vi "HFRR ADV v05 new software.vi"() -> ()   [LabVIEW 2025] (continued)
              }
              frame True {
                w1615 = FALSE ("FRICVALZ")
                n1291 = local write "FRICVALZ 3"(w1615) -> ()
                n1292 = local write "FRICVALZ 2"(w1615) -> ()
                n1293 = local write "FRICVALZ 4"(w1615) -> ()
                "FRICVALZ" <- w1616
              }
            }
            n1294 = Not A Number/Path/Refnum?(number/path/refnum=w1609) -> (NaN/Path/Refnum?=w1608:bool)
            n1295 = Not A Number/Path/Refnum?(number/path/refnum=w1605) -> (NaN/Path/Refnum?=w1607:bool)
            n1296 = Divide(x=w1605, y=1.96) -> (x/y=w1602:dbl)
            n1297 = Compound Arithmetic op=OR(w1608, w1607) -> (w1606:bool)
            n1298 = Not A Number/Path/Refnum?(number/path/refnum=w1602) -> (NaN/Path/Refnum?=w1603:bool)
            n1299 = case shown="True" w1606 {
              frame False {
              }
              frame True {
                n1300 = local write "TEMP"(0.0 ("TEMP")) -> ()
                n1301 = local write "FF 2"(0.0 ("FF 2")) -> ()
                n1302 = local write "reinit"(TRUE ("reinit")) -> ()
              }
            }
            n1303 = Select(t=0.0, s=w1603, f=w1602) -> (s? t:f=w1593:dbl)
            "COF 2" <- w1593
            n1304 = local write "COF 3"(w1593) -> ()
          }
        }
      }
    }
    n1305 = Wait (ms)(milliseconds to wait=u32 50) -> ()  [unwired: 1 out]
    n1306 = local read "Quit"() -> (w1531:bool)
    "Rate" <- 2500.0 ("No of Samples")
  }
  n1307 = while {
    tunnel: w57 -> [_]
    tunnel: [w1643] -> _
    tunnel: [w1619] -> w56
    i -> [w1643]
    stop <- w1619 stop-if-true
    # "C:\\LAB-IQ-NXT\\Scar View.exe"
    n1308 = local read "OK Button 16"() -> (w1632:bool)
    n1309 = local read "Main Tab"() -> (w1625:T2)
    n1310 = local read "service 3"() -> (w1626:bool)
    n1311 = local read "OPEN 6"() -> (w1628:bool)
    n1312 = local read "EDIT 2"() -> (w1630:bool)
    n1313 = flat-sequence {
      frame #0 {
        n1314 = local read "SAVE 2"() -> (w2245:bool)
        n1315 = stacked-sequence {
          frame #0 {
            n1316 = local read "EDIT"() -> (w2299:bool)
            n1317 = case shown="True" w2299 {
              tunnel: [u8 2 ("Disabled") u8 0 ("Disabled")] -> _
              frame False {
                w2301 = FALSE
                n1318 = local write "Password"("") -> ()
                n1319 = property on="SrvM CP" class="Bool (strict)"("Visible"=w2301) -> ()  [unwired: 2 in, 2 out]
                n1320 = property on="message" class="Str"("Visible"=w2301) -> ()  [unwired: 2 in, 2 out]
                n1321 = local write "x = y?"(w2301) -> ()
                n1322 = property on="Password" class="Str"("Visible"=w2301) -> ()  [unwired: 2 in, 2 out]
                n1323 = property on="ENTER THE NEW PASSWORD" class="Str"("Visible"=w2301) -> ()  [unwired: 2 in, 2 out]
                n1324 = property on="ENTER CURRENT PASSWORD" class="Str"("Visible"=w2301) -> ()  [unwired: 2 in, 2 out]
                n1325 = local write "SrvM CP"(w2301) -> ()
              }
              frame True {
                w2304 = TRUE
                n1326 = property on="SrvM CP" class="Bool (strict)"("Visible"=w2304) -> ()  [unwired: 2 in, 2 out]
                n1327 = property on="Password" class="Str"("Visible"=w2304) -> ()  [unwired: 2 in, 2 out]
              }
            }
            "dipl pwd" <- "@143$\n" ("dipl pwd")
          }
          frame #1 {
            # "Gain password"
            n1328 = String To Byte Array(string="ENTER CURRENT PASSWORD") -> (unsigned byte array=w2309:u8[])
            n1329 = Search 1D Array(1D array=w2309, element=u8 10) -> (index of element=w2312:i32)  [unwired: 1 in]
            n1330 = Index Array(array=w2309, index=w2312) -> (element=w2308:u8)
            n1331 = Equal?(x=w2308, y=10) -> (x = y?=w2306:bool)
            n1332 = case shown="True" w2306 {
              frame False {
                n1333 = property on="ENTER THE NEW PASSWORD" class="Str"("Visible"=FALSE) -> ()  [unwired: 2 in, 2 out]
              }
              frame True {
                # "password"
                # "change password logic"
                n1334 = local read "ENTER CURRENT PASSWORD"() -> (w2325:string)
                n1335 = local read "dipl pwd"() -> (w2319:string)
                n1336 = String To Byte Array(string=w2325) -> (unsigned byte array=w2327:u8[])
                n1337 = String To Byte Array(string=w2319) -> (unsigned byte array=w2320:u8[])
                n1338 = Array Size(array=w2327) -> (size(s)=w2324:i32)
                n1339 = Array Size(array=w2320) -> (size(s)=w2322:i32)
                n1340 = for {
                  N: w2324 -> [_]
                  tunnel: w2327 -> [w2351]
                  tunnel: [w2349] -> w2328 mode=indexing
                  tunnel: w2324 -> [w2343]
                  i -> [w2344]
                  n1341 = Decrement(x=w2343) -> (x-1=w2341:i32)
                  n1342 = Equal?(x=w2344, y=w2341) -> (x = y?=w2342:bool)
                  n1343 = Index Array(array=w2351, index=w2344) -> (element=w2345:u8)
                  n1344 = Number To Decimal String(number=w2345) -> (decimal integer string=w2350:string)  [unwired: 1 in]
                  n1345 = Select(t="", s=w2342, f="\r") -> (s? t:f=w2347:string)
                  n1346 = Concatenate Strings(w2350, w2347) -> (w2349:string)
                }
                n1347 = for {
                  N: w2322 -> [_]
                  tunnel: w2320 -> [w2339]
                  tunnel: [w2337] -> w2321 mode=indexing
                  tunnel: w2322 -> [w2334]
                  i -> [w2335]
                  n1348 = Decrement(x=w2334) -> (x-1=w2333:i32)
                  n1349 = Equal?(x=w2335, y=w2333) -> (x = y?=w2332:bool)
                  n1350 = Index Array(array=w2339, index=w2335) -> (element=w2338:u8)
                  n1351 = Number To Decimal String(number=w2338) -> (decimal integer string=w2336:string)  [unwired: 1 in]
                  n1352 = Select(t="", s=w2332, f="\r") -> (s? t:f=w2329:string)
                  n1353 = Concatenate Strings(w2336, w2329) -> (w2337:string)
                }
                n1354 = local read "string"() -> (w2326:string)
                n1355 = Concatenate Strings(w2321) -> (w2315:string)
                n1356 = Concatenate Strings(w2326) -> (w2323:string)
                n1357 = Concatenate Strings(w2328) -> (w2316:string)
                n1358 = Equal?(x=w2316, y=w2323) -> (x = y?=w2318:bool)
                n1359 = Equal?(x=w2316, y=w2315) -> (x = y?=w2314:bool)
                n1360 = Or(x=w2318, y=w2314) -> (x .or. y?=w2317:bool)
                n1361 = case shown="True" w2317 {
                  frame False {
                  }
                  frame True {
                    n1362 = property on="ENTER THE NEW PASSWORD" class="Str"("Visible"=TRUE) -> ()  [unwired: 2 in, 2 out]
                  }
                }
              }
            }
          }
          frame #2 {
            n1363 = String To Byte Array(string="ENTER THE NEW PASSWORD") -> (unsigned byte array=w2354:u8[])
            n1364 = Search 1D Array(1D array=w2354, element=u8 10) -> (index of element=w2358:i32)  [unwired: 1 in]
            n1365 = Index Array(array=w2354, index=w2358) -> (element=w2356:u8)
            n1366 = Equal?(x=w2356, y=10) -> (x = y?=w2353:bool)
            n1367 = case shown="False" w2353 {
              frame False {
              }
              frame True {
                n1368 = local write "EDIT"(FALSE) -> ()
                n1369 = local write "SrvM CP"(FALSE) -> ()
                n1370 = local read "ENTER THE NEW PASSWORD"() -> (w2361:string)
                n1371 = String To Byte Array(string=w2361) -> (unsigned byte array=w2366:u8[])
                n1372 = Array Size(array=w2366) -> (size(s)=w2363:i32)
                n1373 = for {
                  N: w2363 -> [_]
                  tunnel: w2366 -> [w2379]
                  tunnel: [w2376] -> w2368 mode=indexing
                  tunnel: w2363 -> [w2371]
                  i -> [w2369]
                  n1374 = Decrement(x=w2371) -> (x-1=w2372:i32)
                  n1375 = Equal?(x=w2369, y=w2372) -> (x = y?=w2373:bool)
                  n1376 = Index Array(array=w2379, index=w2369) -> (element=w2378:u8)
                  n1377 = Number To Decimal String(number=w2378) -> (decimal integer string=w2377:string)  [unwired: 1 in]
                  n1378 = Select(t="", s=w2373, f="\r") -> (s? t:f=w2370:string)
                  n1379 = Concatenate Strings(w2377, w2370) -> (w2376:string)
                }
                n1380 = local read "file path"() -> (w2360:path)
                n1381 = Concatenate Strings(w2368) -> (w2362:string)
                n1382 = Delete(path (use dialog)=w2360) -> (deleted path=w2364:path)  [unwired: 4 in, 2 out]
                n1383 = call <vilib>:"Write Characters To File.vi"("append to file? (new file:F)"=FALSE, "character string"=w2362, "file path (dialog if empty)"=w2364) -> ()  [unwired: 2 in, 1 out]
              }
            }
          }
          frame #3 {
            n1384 = case shown="True" "SrvM CP" {
              frame False {
                w2382 = ""
                n1385 = local write "ENTER CURRENT PASSWORD"(w2382) -> ()
                n1386 = local write "ENTER THE NEW PASSWORD"(w2382) -> ()
                n1387 = property on="ENTER CURRENT PASSWORD" class="Str"("Visible"=FALSE) -> ()  [unwired: 2 in, 2 out]
              }
              frame True {
                n1388 = property on="ENTER THE NEW PASSWORD" class="Str"() -> ("Visible"=w2383:bool)  [unwired: 2 in, 2 out]
                n1389 = Not(x=w2383) -> (.not. x?=w2384:bool)
                n1390 = property on="ENTER CURRENT PASSWORD" class="Str"("Visible"=w2384) -> ()  [unwired: 2 in, 2 out]
              }
            }
          }
          frame #4 {
            n1391 = String To Byte Array(string="Password") -> (unsigned byte array=w2391:u8[])
            n1392 = Search 1D Array(1D array=w2391, element=u8 10) -> (index of element=w2389:i32)  [unwired: 1 in]
            n1393 = Index Array(array=w2391, index=w2389) -> (element=w2390:u8)
            n1394 = Equal?(x=w2390, y=10) -> (x = y?=w2386:bool)
            n1395 = case shown="True" w2386 {
              frame False {
              }
              frame True {
                # "password"
                # "password"
                n1396 = local read "Password"() -> (w2404:string)
                n1397 = String To Byte Array(string=w2404) -> (unsigned byte array=w2407:u8[])
                n1398 = String To Byte Array(string="@143$\n") -> (unsigned byte array=w2393:u8[])
                n1399 = Array Size(array=w2407) -> (size(s)=w2402:i32)
                n1400 = Array Size(array=w2393) -> (size(s)=w2398:i32)
                n1401 = for {
                  N: w2402 -> [_]
                  tunnel: w2407 -> [w2441]
                  tunnel: [w2439] -> w2408 mode=indexing
                  tunnel: w2402 -> [w2436]
                  i -> [w2437]
                  n1402 = Decrement(x=w2436) -> (x-1=w2435:i32)
                  n1403 = Index Array(array=w2441, index=w2437) -> (element=w2440:u8)
                  n1404 = Equal?(x=w2437, y=w2435) -> (x = y?=w2434:bool)
                  n1405 = Number To Decimal String(number=w2440) -> (decimal integer string=w2438:string)  [unwired: 1 in]
                  n1406 = Select(t="", s=w2434, f="\r") -> (s? t:f=w2431:string)
                  n1407 = Concatenate Strings(w2438, w2431) -> (w2439:string)
                }
                n1408 = for {
                  N: w2398 -> [_]
                  tunnel: w2393 -> [w2452]
                  tunnel: [w2450] -> w2396 mode=indexing
                  tunnel: w2398 -> [w2447]
                  i -> [w2448]
                  n1409 = Decrement(x=w2447) -> (x-1=w2446:i32)
                  n1410 = Index Array(array=w2452, index=w2448) -> (element=w2451:u8)
                  n1411 = Equal?(x=w2448, y=w2446) -> (x = y?=w2445:bool)
                  n1412 = Number To Decimal String(number=w2451) -> (decimal integer string=w2449:string)  [unwired: 1 in]
                  n1413 = Select(t="", s=w2445, f="\r") -> (s? t:f=w2442:string)
                  n1414 = Concatenate Strings(w2449, w2442) -> (w2450:string)
                }
                n1415 = local read "file path"() -> (w2392:path)
                n1416 = call <vilib>:"Read Characters From File.vi"("file path (dialog if empty)"=w2392) -> ("character string"=w2406:string)  [unwired: 5 in, 3 out]
                "string" <- w2406
                n1417 = flat-sequence {
                  tunnel: [w2409] -> w2403
                  frame #0 {
                    w2409 = ""
                    n1418 = local write "Password"(w2409) -> ()
                  }
                }
                n1419 = Concatenate Strings(w2396) -> (w2397:string)
                n1420 = Concatenate Strings(w2406) -> (w2405:string)
                n1421 = Concatenate Strings(w2408) -> (w2400:string)
                n1422 = Equal?(x=w2400, y=w2405) -> (x = y?=w2395:bool)
                n1423 = Equal?(x=w2400, y=w2397) -> (x = y?=w2401:bool)
                n1424 = Or(x=w2395, y=w2401) -> (x .or. y?=w2394:bool)
                "x = y?" <- w2394
                n1425 = case shown="True" w2394 {
                  selector: w2394 -> [w2411 _]
                  tunnel: w2403 -> [_ _]
                  frame False {
                    n1426 = And(x=w2411, y=TRUE ("Visible")) -> (x .and. y?=w2412:bool)
                    n1427 = property on="message" class="Str"("Visible"=w2412) -> ()  [unwired: 2 in, 2 out]
                  }
                  frame True {
                    n1428 = control-ref of="This VI"() -> (w2423:refnum<vi>)
                    n1429 = property class="VI"(reference=w2423) -> (reference out=w2414:refnum<vi>, error out=w2418:errorcluster, "Panel"=w2422:refnum<vi>)  [unwired: 1 in]
                    n1430 = property on="message" class="Str"("Visible"=FALSE) -> ()  [unwired: 2 in, 2 out]
                    n1431 = property class="Pnl"(reference=w2422, error in=w2418) -> (reference out=w2416:refnum<vi>, error out=w2419:errorcluster, "Panes[]"=w2421:refnum<vi>[])
                    n1432 = for {
                      tunnel: w2421 -> [w2430] mode=indexing
                      tunnel: T15."Always On" ("Horizontal Scrollbar Visibility") -> [w2429]
                      tunnel: w2419 -> [w2426]
                      tunnel: [w2425] -> w2417
                      n1433 = property class="Pane"(reference=w2430, error in=w2426, "HorizScrollbarVisibility"=w2429) -> (reference out=w2427:refnum<vi>, error out=w2428:errorcluster)
                      n1434 = Close Reference(reference=w2427, error in (no error)=w2428) -> (error out=w2425:errorcluster)
                    }
                    n1435 = Close Reference(reference=w2416, error in (no error)=w2417) -> (error out=w2415:errorcluster)
                    n1436 = Close Reference(reference=w2414, error in (no error)=w2415) -> (error out=→"error out 6":errorcluster)
                  }
                }
              }
            }
          }
        }
        n1437 = local read "x = y?"() -> (w2251:bool)
        n1438 = local read "HUMIDITY: 2"() -> (w2253:dbl)
        n1439 = local read "HUMIDITY:"() -> (w2252:dbl)
        n1440 = property on="Port 2 Error" class="Clust (strict)"("Visible"="EDIT") -> ()  [unwired: 2 in, 2 out]
        n1441 = property on="Port 1 Error" class="Clust (strict)"("Visible"="EDIT") -> ()  [unwired: 2 in, 2 out]
        n1442 = case shown="True" "SrvM CP 2" {
          frame False {
          }
          frame True {
            n1443 = local write "SrvM CP 2"(FALSE ("SrvM CP 2")) -> ()
            n1444 = local read "HUMIDITY: 2"() -> (w2292:dbl)
            n1445 = local read "TEMP INTERCEPT: 2"() -> (w2291:dbl)
            n1446 = local read "DISPLACEMENT : 4"() -> (w2295:dbl)
            n1447 = local read "TEMPERATURE : 2"() -> (w2294:dbl)
            n1448 = local read "STROKE GAIN : 2"() -> (w2296:dbl)
            n1449 = local read "FRIC. FORCE : 2"() -> (w2297:dbl)
            n1450 = local read "AIR TEMP INTERCEPT: 2"() -> (w2290:dbl)
            n1451 = local read "AIR TEMPERATURE : 2"() -> (w2293:dbl)
            n1452 = local write "HUMIDITY:"(w2292) -> ()
            n1453 = local write "AIR TEMP INTERCEPT:"(w2291) -> ()
            n1454 = local write "TEMPERATURE :"(w2294) -> ()
            n1455 = local write "FRIC. FORCE :"(w2297) -> ()
            n1456 = local write "STROKE GAIN :"(w2296) -> ()
            n1457 = local write "DISPLACEMENT :"(w2295) -> ()
            n1458 = local write "AIR TEMPERATURE :"(w2293) -> ()
            n1459 = local write "TEMP INTERCEPT:"(w2290) -> ()
          }
        }
        n1460 = Or(x="SAVE", y=w2245) -> (x .or. y?=w2246:bool)
        n1461 = And(x="EDIT", y=w2251) -> (x .and. y?=w2249:bool)
        n1462 = local read "DISPLACEMENT : 4"() -> (w2262:dbl)
        n1463 = local read "TEMPERATURE : 2"() -> (w2260:dbl)
        n1464 = local read "STROKE GAIN : 2"() -> (w2266:dbl)
        n1465 = local read "DISPLACEMENT :"() -> (w2261:dbl)
        n1466 = local read "FRIC. FORCE : 2"() -> (w2269:dbl)
        n1467 = local read "TEMPERATURE :"() -> (w2258:dbl)
        n1468 = local read "STROKE GAIN :"() -> (w2265:dbl)
        n1469 = local read "FRIC. FORCE :"() -> (w2268:dbl)
        n1470 = case shown="True" w2249 {
          tunnel: [u8 2 ("Disabled") u8 0 ("Disabled")] -> w2248
          tunnel: [w2613 TRUE ("Visible")] -> w2247
          frame False {
            w2613 = FALSE ("Visible")
            n1471 = local write "EDIT 2"(w2613) -> ()
          }
          frame True {
          }
        }
        n1472 = case shown="True" w2246 {
          frame False {
          }
          frame True {
            n1473 = stacked-sequence {
              seq-local: [w2461 _ _] -> [_ w2608 _]
              frame #0 {
                (unwired) i16 5 ("precision (6)")
                # "[CH1]    - FF\n[CH2]   - TEMPERATURE\n[CH3]    - Humidity\n[CH4]    - AIR TEMP\n[CH5]\\- Visa Uno\n[CH6] \\- Visa Due\n[CH7]  \\- file path\n[CH8]   - Displacement Gain\n[CHA]   - Stroke Gain\n[CHB]   - Stroke PID Gain\n[CHC]   -Language Selection\n[CHD]   -Power +\n[CHE]   -Power_\n[CHF]   -Heater\n[CHG]   -Humidity Wet\n[CHH]   -Humidity Dry\n[CHI]   -Integral Time"
                n1474 = local read "Language Selection"() -> (w2509:enum16{"English", "Russian"})
                n1475 = local read "CH-HUMIDITY WET"() -> (w2467:u16)
                n1476 = local read "CH-HUMIDITY DRY"() -> (w2464:u16)
                n1477 = local read "STROKE GAIN :"() -> (w2453:dbl)
                n1478 = local read "CH-POWER +"() -> (w2476:u16)
                n1479 = local read "CH-POWER -"() -> (w2473:u16)
                n1480 = local read "CH-HEATER"() -> (w2470:u16)
                n1481 = local read "AIR TEMPERATURE :"() -> (w2456:dbl)
                n1482 = local read "DISPLACEMENT :"() -> (w2454:dbl)
                n1483 = local read "TEMPERATURE :"() -> (w2457:dbl)
                n1484 = local read "FRIC. FORCE :"() -> (w2458:dbl)
                n1485 = local read "HUMIDITY:"() -> (w2455:dbl)
                n1486 = Path To String(path="File Path") -> (string=w2525:string)
                n1487 = Number To Fractional String(number=w2453, width (-)=i16 10 ("precision (6)"), precision (6)=i16 5) -> (F-format string=w2516:string)  [unwired: 1 in]
                n1488 = Number To Fractional String(number=w2509, width (-)=i16 10 ("precision (6)"), precision (6)=i16 5) -> (F-format string=w2505:string)  [unwired: 1 in]
                n1489 = Number To Fractional String(number=w2476, width (-)=i16 10 ("precision (6)"), precision (6)=i16 5) -> (F-format string=w2499:string)  [unwired: 1 in]
                n1490 = Number To Fractional String(number=w2473, width (-)=i16 10 ("precision (6)"), precision (6)=i16 5) -> (F-format string=w2496:string)  [unwired: 1 in]
                n1491 = Number To Fractional String(number=w2470, width (-)=i16 10 ("precision (6)"), precision (6)=i16 5) -> (F-format string=w2491:string)  [unwired: 1 in]
                n1492 = Number To Fractional String(number=w2467, width (-)=i16 10 ("precision (6)"), precision (6)=i16 5) -> (F-format string=w2488:string)  [unwired: 1 in]
                n1493 = Number To Fractional String(number=w2464, width (-)=i16 10 ("precision (6)"), precision (6)=i16 5) -> (F-format string=w2483:string)  [unwired: 1 in]
                n1494 = local read "Com Port 1"() -> (w2460:refnum<visa-resource-name>)
                n1495 = local read "Com Port 2"() -> (w2459:refnum<visa-resource-name>)
                n1496 = Concatenate Strings(w2525, "\\" ("string")) -> (w2524:string)
                n1497 = Number To Fractional String(number=w2458, width (-)=i16 10 ("precision (6)"), precision (6)=i16 5) -> (F-format string=w2557:string)  [unwired: 1 in]
                n1498 = Number To Fractional String(number=w2457, width (-)=i16 10 ("precision (6)"), precision (6)=i16 5) -> (F-format string=w2556:string)  [unwired: 1 in]
                n1499 = Number To Fractional String(number=w2455, width (-)=i16 10 ("precision (6)"), precision (6)=i16 5) -> (F-format string=w2550:string)  [unwired: 1 in]
                n1500 = Number To Fractional String(number=w2456, width (-)=i16 10 ("precision (6)"), precision (6)=i16 5) -> (F-format string=w2544:string)  [unwired: 1 in]
                n1501 = Number To Fractional String(number=w2454, width (-)=i16 10 ("precision (6)"), precision (6)=i16 5) -> (F-format string=w2517:string)  [unwired: 1 in]
                n1502 = Concatenate Strings("[CHA]" ("string"), w2516, "- Stroke Gain" ("string"), "\r") -> (w2510:string)
                n1503 = Concatenate Strings("[CHC]" ("string"), w2505, "-Language Selection" ("string"), "\r") -> (w2502:string)
                n1504 = Concatenate Strings("[CHD]" ("string"), w2499, "-Power +" ("string"), "\r") -> (w2481:string)
                n1505 = Concatenate Strings("[CHG]" ("string"), w2488, "-Humidity Wet" ("string"), "\r") -> (w2478:string)
                n1506 = Concatenate Strings("[CHH]" ("string"), w2483, "-Humidity Dry" ("string"), "\r") -> (w2477:string)
                n1507 = Concatenate Strings("[CH1]" ("string"), w2557, " - FF" ("string"), "\r") -> (w2555:string)
                n1508 = Concatenate Strings("[CH2]" ("string"), w2556, " - TEMPERATURE" ("string"), "\r") -> (w2554:string)
                n1509 = Concatenate Strings("[CH3]" ("string"), w2550, " - Humidity" ("string"), "\r") -> (w2547:string)
                n1510 = Concatenate Strings("[CH4]" ("string"), w2544, " - AIR TEMP" ("string"), "\r") -> (w2540:string)
                n1511 = Concatenate Strings("[CH5]" ("string"), w2460, "- Visa Uno" ("string"), "\r") -> (w2533:string)
                n1512 = Concatenate Strings("[CH6]" ("string"), w2459, "- Visa Due" ("string"), "\r") -> (w2528:string)
                n1513 = Concatenate Strings("[CH7]" ("string"), w2524, "- file path" ("string"), "\r") -> (w2527:string)
                n1514 = Concatenate Strings("[CH8]" ("string"), w2517, "- Displacement Gain" ("string"), "\r") -> (w2520:string)
                n1515 = Concatenate Strings("[CHE]" ("string"), w2496, "-Power_" ("string"), "\r") -> (w2480:string)
                n1516 = Concatenate Strings("[CHF]" ("string"), w2491, "-Heater" ("string"), "\r") -> (w2479:string)
                n1517 = Concatenate Strings(w2555, w2554, w2547, w2540, w2533, w2528, w2527, w2520, w2510, w2502, w2481, w2480, w2479, w2478, w2477) -> (w2461:string)
                "gain" <- w2461
              }
              frame #1 {
                n1518 = local read "Camera Port :"() -> (w2569:string)
                n1519 = local read "C3 :"() -> (w2577:refnum<visa-resource-name>)
                n1520 = local read "TEMP INTERCEPT:"() -> (w2578:dbl)
                n1521 = local read "AIR TEMP INTERCEPT:"() -> (w2579:dbl)
                n1522 = Concatenate Strings("[CH8]" ("string"), w2569, "- Visa Camera" ("string"), "\r") -> (w2568:string)
                n1523 = Concatenate Strings("[CH7]" ("string"), w2577, "- Visa Humidity" ("string"), "\r") -> (w2573:string)
                n1524 = Number To Fractional String(number=w2578, width (-)=i16 10 ("precision (6)"), precision (6)=i16 5) -> (F-format string=w2596:string)  [unwired: 1 in]
                n1525 = local read "Com Port 3"() -> (w2580:refnum<visa-resource-name>)
                n1526 = Number To Fractional String(number=w2579, width (-)=i16 10 ("precision (6)"), precision (6)=i16 5) -> (F-format string=w2603:string)  [unwired: 1 in]
                n1527 = Concatenate Strings("[CHK]" ("string"), w2596, "-TEMP INTERCEPT" ("string"), "\r") -> (w2592:string)
                n1528 = Concatenate Strings("[SNO]" ("string"), "S.NO", "-" ("string"), "\r") -> (w2588:string)
                n1529 = Concatenate Strings("[CHJ]" ("string"), w2603, "-AIR TEMP INTERCEPT" ("string"), "\r") -> (w2593:string)
                n1530 = Concatenate Strings("[CHL]" ("string"), w2580, "- Visa humid" ("string"), "\r") -> (w2583:string)
                n1531 = String To Path(string="C:\\LAB-IQ\\calibrate WO 2465.dcf") -> (path=w2581:path)
                n1532 = Concatenate Strings(w2608, w2593, w2592, w2588, w2583, w2573, w2568) -> (w2607:string)
                n1533 = call <vilib>:"Write Characters To File.vi"("append to file? (new file:F)"=FALSE, "character string"=w2607, "file path (dialog if empty)"=w2581) -> ()  [unwired: 2 in, 1 out]
              }
              frame #2 {
                n1534 = local write "Lan flag"(0.0 ("Lan flag")) -> ()
                n1535 = local write "conststatus"(0.0 ("rpm value : 2")) -> ()
                n1536 = local write "SAVE"(FALSE ("OK Button 14")) -> ()
                n1537 = local write "SAVE 2"(FALSE ("SAVE 2")) -> ()
              }
            }
          }
        }
        n1538 = Subtract(x=w2253, y=w2252) -> (x-y=w2254:dbl)
        n1539 = local read "AIR TEMPERATURE : 2"() -> (w2257:dbl)
        n1540 = local read "AIR TEMPERATURE :"() -> (w2256:dbl)
        n1541 = Divide(x=w2254, y=w2252) -> (x/y=w2276:dbl)
        n1542 = Subtract(x=w2269, y=w2268) -> (x-y=w2267:dbl)
        n1543 = Subtract(x=w2260, y=w2258) -> (x-y=w2259:dbl)
        n1544 = Subtract(x=w2266, y=w2265) -> (x-y=w2264:dbl)
        n1545 = Subtract(x=w2262, y=w2261) -> (x-y=w2263:dbl)
        n1546 = Subtract(x=w2257, y=w2256) -> (x-y=w2255:dbl)
        n1547 = Divide(x=w2267, y=w2268) -> (x/y=w2287:dbl)
        n1548 = Divide(x=w2259, y=w2258) -> (x/y=w2280:dbl)
        n1549 = Divide(x=w2264, y=w2265) -> (x/y=w2284:dbl)
        n1550 = Divide(x=w2263, y=w2261) -> (x/y=w2283:dbl)
        n1551 = Multiply(x=w2276, y=100.0) -> (x*y=→"HUMIDITY  Calibration Error":dbl)
        n1552 = Divide(x=w2255, y=w2256) -> (x/y=w2279:dbl)
        n1553 = Multiply(x=w2287, y=100.0) -> (x*y=→"FRIC. FORCE Calibration Error":dbl)
        n1554 = Multiply(x=w2280, y=100.0) -> (x*y=→"TEMPERATURE  Calibration Error":dbl)
        n1555 = Multiply(x=w2284, y=100.0) -> (x*y=→"STROKE Calibration Error":dbl)
        n1556 = Multiply(x=w2283, y=100.0) -> (x*y=→"DISPLACEMENT  Calibration Error":dbl)
        n1557 = property on="EDIT 2" class="Bool (strict)"("Visible"=w2247) -> ()  [unwired: 2 in, 2 out]
        n1558 = property on="SAVE" class="Bool (strict)"("Visible"=w2247) -> ()  [unwired: 2 in, 2 out]
        n1559 = property on="SrvM CP" class="Bool (strict)"("Disabled"=w2248) -> ()  [unwired: 2 in, 2 out]
        n1560 = property on="visa due" class="CmbBox"("Disabled"=w2248) -> ()  [unwired: 2 in, 2 out]
        n1561 = property on="File Path" class="Path"("Disabled"=w2248) -> ()  [unwired: 2 in, 2 out]
        n1562 = Multiply(x=w2279, y=100.0) -> (x*y=→"AIR TEMPERATURE  Calibration Error":dbl)
        n1563 = property on="Language Selection" class="Enum (strict)"("Visible"=w2247) -> ()  [unwired: 2 in, 2 out]
        n1564 = property on="Tab Control 7" class="TabCtl (strict)"("Disabled"=w2248) -> ()  [unwired: 2 in, 2 out]
        n1565 = property on="AIR TEMP INTERCEPT:" class="DigNum (strict)"("Disabled"=w2248) -> ()  [unwired: 2 in, 2 out]
        n1566 = property on="CH-POWER -" class="DigNum (strict)"("Disabled"=w2248) -> ()  [unwired: 2 in, 2 out]
        n1567 = property on="CH-POWER +" class="DigNum (strict)"("Disabled"=w2248) -> ()  [unwired: 2 in, 2 out]
        n1568 = property on="AIR TEMPERATURE :" class="DigNum (strict)"("Disabled"=w2248) -> ()  [unwired: 2 in, 2 out]
        n1569 = property on="STROKE GAIN :" class="DigNum (strict)"("Disabled"=w2248) -> ()  [unwired: 2 in, 2 out]
        n1570 = property on="SPEED OUT:" class="DigNum (strict)"("Disabled"=w2248) -> ()  [unwired: 2 in, 2 out]
        n1571 = property on="CH-HUMIDITY DRY" class="DigNum (strict)"("Disabled"=w2248) -> ()  [unwired: 2 in, 2 out]
        n1572 = property on="HUMIDITY:" class="DigNum (strict)"("Disabled"=w2248) -> ()  [unwired: 2 in, 2 out]
        n1573 = property on="CH-HUMIDITY WET" class="DigNum (strict)"("Disabled"=w2248) -> ()  [unwired: 2 in, 2 out]
        n1574 = property on="TEMPERATURE :" class="DigNum (strict)"("Disabled"=w2248) -> ()  [unwired: 2 in, 2 out]
        n1575 = property on="DISPLACEMENT :" class="DigNum (strict)"("Disabled"=w2248) -> ()  [unwired: 2 in, 2 out]
        n1576 = property on="CH-HEATER" class="DigNum (strict)"("Disabled"=w2248) -> ()  [unwired: 2 in, 2 out]
        n1577 = property on="TEMP INTERCEPT:" class="DigNum (strict)"("Disabled"=w2248) -> ()  [unwired: 2 in, 2 out]
        n1578 = property on="FRIC. FORCE :" class="DigNum (strict)"("Disabled"=w2248) -> ()  [unwired: 2 in, 2 out]
      }
    }
    n1579 = local read "RUN"() -> (w1642:bool)
    n1580 = local read "RUN"() -> (w1640:bool)
    n1581 = disable-structure shown="Disabled" {
      disable-tunnel: [w1657 _] -> w1623
      disable-tunnel: [w1656 _] -> w1621
      frame Disabled {
        n1582 = local read "Temperature before test"() -> (w1650:dbl)
        n1583 = local read "Temperature after test"() -> (w1663:dbl)
        n1584 = case shown="True" "Save Results" {
          frame False {
          }
          frame True {
            w1679 = "\r"
            n1585 = local write "Save Results"(FALSE ("OK Button 5")) -> ()
            n1586 = local read "Temperature before test"() -> (w1717:dbl)
            n1587 = local read "Temperature after test"() -> (w1719:dbl)
            n1588 = local read "Humidity before test"() -> (w1716:dbl)
            n1589 = local read "Humidity after test"() -> (w1718:dbl)
            n1590 = local read "WS1.4"() -> (w1723:dbl)
            n1591 = local read "AVP"() -> (w1721:dbl)
            n1592 = Number To Fractional String(number=w1723, width (-)=i16 6, precision (6)=i16 1) -> (F-format string=w1683:string)  [unwired: 1 in]
            n1593 = local read "MWSD"() -> (w1720:dbl)
            n1594 = local read "String"() -> (w1712:string)
            n1595 = local read "FILE"() -> (w1715:string)
            n1596 = local read "HCF"() -> (w1722:dbl)
            n1597 = Number To Fractional String(number=w1716, width (-)=i16 6, precision (6)=i16 1) -> (F-format string=w1708:string)  [unwired: 1 in]
            n1598 = Number To Fractional String(number=w1717, width (-)=i16 6, precision (6)=i16 1) -> (F-format string=w1705:string)  [unwired: 1 in]
            n1599 = Number To Fractional String(number=w1718, width (-)=i16 6, precision (6)=i16 1) -> (F-format string=w1701:string)  [unwired: 1 in]
            n1600 = Number To Fractional String(number=w1719, width (-)=i16 6, precision (6)=i16 1) -> (F-format string=w1697:string)  [unwired: 1 in]
            n1601 = Number To Fractional String(number=w1721, width (-)=i16 6, precision (6)=i16 3) -> (F-format string=w1690:string)  [unwired: 1 in]
            n1602 = Concatenate Strings(w1712, w1715) -> (w1734:string)
            n1603 = Number To Fractional String(number=w1720, width (-)=i16 6, precision (6)=i16 1) -> (F-format string=w1694:string)  [unwired: 1 in]
            n1604 = Number To Fractional String(number=w1722, width (-)=i16 6, precision (6)=i16 2) -> (F-format string=w1688:string)  [unwired: 1 in]
            n1605 = Concatenate Strings("(" ("string"), w1683, ")Microns" ("string")) -> (w1682:string)
            n1606 = local read "REMARKS"() -> (w1714:string)
            "REMARKS 2" <- w1714
            n1607 = Concatenate Strings("(" ("string"), w1708, " ) % RH," ("string")) -> (w1709:string)
            n1608 = Concatenate Strings(w1688, ")" ("string")) -> (w1686:string)
            n1609 = Concatenate Strings("(" ("string"), w1705, ")  Deg C ," ("string")) -> (w1704:string)
            n1610 = Concatenate Strings("(" ("string"), w1701, " ) % RH," ("string")) -> (w1700:string)
            n1611 = Concatenate Strings("(" ("string"), w1697, ")  Deg C ," ("string")) -> (w1696:string)
            n1612 = Concatenate Strings("(" ("string"), w1694, ")  Microns," ("string")) -> (w1693:string)
            n1613 = Concatenate Strings("(" ("string"), w1690, ")  kPa," ("string")) -> (w1680:string)
            n1614 = Concatenate Strings(w1734, ".dwm" ("Substring")) -> (w1732:string)
            n1615 = String To Path(string=w1732) -> (path=w1731:path)
            n1616 = Concatenate Strings(w1714, w1679, " Humidity before test= " ("Substring"), w1709, w1679, " Temperature before test = " ("Substring"), w1704, w1679, " Humidity after test= " ("Substring"), w1700, w1679, "Temperature after test = " ("Substring"), w1696, w1679, "MSD = " ("Substring"), w1693, w1679, "  AVP = " ("Substring"), w1680, w1679, "  HCF                     =( " ("Substring"), w1686, w1679, " WS1.4                  = " ("Substring"), w1682, w1679) -> (w1678:string)
            "data" <- w1678
            n1617 = call <vilib>:"Write Characters To File.vi"("append to file? (new file:F)"=FALSE, "character string"=w1678, "file path (dialog if empty)"=w1731) -> ()  [unwired: 2 in, 1 out]
            n1618 = Match Pattern(string=w1678, regular expression="!") -> (after substring=→"export":string)  [unwired: 1 in, 3 out]
          }
        }
        n1619 = Add(x=231.864, y=w1650) -> (x+y=w1647:dbl)
        n1620 = Add(x=231.864, y=w1663) -> (x+y=w1660:dbl)
        n1621 = Divide(x=1705.984, y=w1647) -> (x/y=w1648:dbl)
        n1622 = Divide(x=1705.984, y=w1660) -> (x/y=w1661:dbl)
        n1623 = local read "Humidity before test"() -> (w1652:dbl)
        n1624 = local read "Humidity after test"() -> (w1665:dbl)
        n1625 = Subtract(x=8.017352 ("y"), y=w1648) -> (x-y=w1674:dbl)
        n1626 = Subtract(x=8.017352 ("y"), y=w1661) -> (x-y=w1668:dbl)
        n1627 = expression code="10**y"(w1674) -> (w1654:dbl)
        n1628 = expression code="10**y"(w1668) -> (w1667:dbl)
        n1629 = Multiply(x=w1652, y=w1654) -> (x*y=w1653:dbl)
        n1630 = Multiply(x=w1665, y=w1667) -> (x*y=w1666:dbl)
        n1631 = Divide(x=w1653, y=750.0) -> (x/y=w1669:dbl)
        n1632 = Divide(x=w1666, y=750.0) -> (x/y=w1670:dbl)
        n1633 = Add(x=w1669, y=w1670) -> (x+y=w1671:dbl)
        n1634 = Divide(x=w1671, y=2.0) -> (x/y=w1673:dbl)
        n1635 = local write "AVP"(w1673) -> ()
        n1636 = Subtract(x=1.4, y=w1673) -> (x-y=w1656:dbl)
        n1637 = local read "HCF"() -> (w1657:dbl)
      }
      frame Enabled {
      }
    }
    n1638 = case shown="True" "EDIT 3" {
      frame False {
      }
      frame True {
        n1639 = local write "EDIT 3"(FALSE ("EDIT 3")) -> ()
        n1640 = local write "Main Tab"(T2."About" ("Main Tab")) -> ()
      }
    }
    n1641 = case shown="False" w1642 {
      frame False {
        n1642 = local read "stopT"() -> (w2620:bool)
        n1643 = case shown="True" w2620 {
          frame False {
          }
          frame True {
            n1644 = local write "stopT"(FALSE) -> ()
          }
        }
      }
      frame True {
        "stopT" <- TRUE
      }
    }
    n1645 = case shown="False" w1640 {
      frame False {
      }
      frame True {
      }
    }
    n1646 = case shown="True" w1630 {
      frame False {
        n1647 = property on="Password 2" class="Str"("Visible"=FALSE) -> ()  [unwired: 2 in, 2 out]
        n1648 = local write "Password 2"("" ("Password")) -> ()
      }
      frame True {
        n1649 = property on="Password 2" class="Str"("Visible"=TRUE) -> ()  [unwired: 2 in, 2 out]
        n1650 = Equal?(x="Password 2", y="HFRR1234") -> (x = y?=w1762:bool)
        n1651 = case shown="True" w1762 {
          tunnel: "Password 2" -> [w1765 _]
          frame False {
            n1652 = String Length(string=w1765) -> (length=w1766:i32)
            n1653 = Greater Than 0?(x=w1766) -> (x > 0?=w1764:bool)
            n1654 = case shown="False" w1764 {
              frame False {
                n1655 = property on="Password 2" class="Str"("Caption.Text"="Password (Advance Setting)") -> ()  [unwired: 2 in, 2 out]
              }
              frame True {
                n1656 = property on="Password 2" class="Str"("Caption.Text"="Incorrect Password!") -> ()  [unwired: 2 in, 2 out]
              }
            }
          }
          frame True {
            n1657 = local write "EDIT 2"(FALSE ("EDIT 2")) -> ()
            n1658 = local write "Password 2"("" ("Password")) -> ()
            n1659 = local write "Main Tab"(T2."Advance" ("Main Tab")) -> ()
            n1660 = local write "Main Dashboard Buttons"(T1."Advance" ("Main Dashboard Buttons")) -> ()
          }
        }
      }
    }
    n1661 = case shown="True" "Prog Uno" {
      frame False {
      }
      frame True {
        n1662 = stacked-sequence {
          frame #0 {
            n1663 = Delete(path (use dialog)=path "C:/LAB-IQ-NXT/UNOCOMPILE.bat" ("working directory")) -> ()  [unwired: 4 in, 3 out]
          }
          frame #1 {
            n1664 = local read "Com Port 1"() -> (w2227:refnum<visa-resource-name>)
            n1665 = Concatenate Strings("cmd.exe /c \"mode " ("command line"), w2227, ":1200,n,8,1\"\n" ("command line")) -> (w2232:string)
            n1666 = Concatenate Strings(w2232, "CD\\\nCD WinDucom\navrdude -C avrdude.conf -v -patmega328p -carduino -P" ("command line"), w2227, " -b115200 -D -Uflash:w:UNO_V20.hex:i\n" ("command line"), "\r") -> (w2234:string)
            "STR" <- w2234
            n1667 = call <vilib>:"Write Characters To File.vi"("append to file? (new file:F)"=FALSE, "character string"=w2234, "file path (dialog if empty)"=path "C:/LAB-IQ/UNOCOMPILE.bat" ("working directory")) -> ()  [unwired: 2 in, 1 out]
          }
          frame #2 {
            n1668 = disable-structure shown="Disabled" {
              frame Disabled {
                w2238 = "cmd.exe  /c \"C:\\LAB-IQ-NXT\\UNOCOMPILE.bat\"" ("string")
                n1669 = local write "Prog Uno"(FALSE ("run minimized? (F)")) -> ()
                n1670 = call <vilib>:"System Exec.vi"("expected output size  (4096)"=u32 65535, "run minimized? (F)"=FALSE, "wait until completion? (T)"=TRUE ("run minimized? (F)"), "working directory"=path "C:/LAB-IQ-NXT", "standard input"=w2238, "command line"=w2238) -> ("error out"=w2237:errorcluster, "standard output"=→"String 42":string)  [unwired: 2 in, 2 out]
                "error out 3" <- w2237
                n1671 = flat-sequence {
                  tunnel: w2237 -> [_]
                  frame #0 {
                  }
                }
              }
              frame Enabled {
              }
            }
          }
        }
      }
    }
    n1672 = case shown="\"CEC F-096-A-06\"" "TEST STANDARD" {
      tunnel: [2.0 ("Set Temp") 0.0 ("Set Temp") 2.0 ("Set Temp") 0.0 ("Set Temp")] -> w1631
      frame "ASTM D6079", Default {
        w2184 = 50.0 ("Hz")
        w2185 = 53.0 ("Set Rh")
        w2187 = 1.0 ("Set Strk")
        w2186 = 60.0 ("Set Temp")
        # "astm hide"
        n1673 = local write "NORMAL LOAD"(200.0 ("NORMAL LOAD")) -> ()
        n1674 = local write "Set Strk"(w2187) -> ()
        n1675 = local write "Set Hz"(w2184) -> ()
        n1676 = local write "Set Temp"(w2186) -> ()
        n1677 = local write "Set Rh"(w2185) -> ()
        n1678 = local write "test time"(75.0 ("test time")) -> ()
        n1679 = local write "Set Stroke:"(w2187) -> ()
        n1680 = local write "Set Humidity:"(w2185) -> ()
        n1681 = local write "Set Frequency:"(w2184) -> ()
        n1682 = local write "Set Temperature:"(w2186) -> ()
        "Test Standard" <- "ASTM D6079" ("Test Standard 2")
      }
      frame "ISO 12156" {
        n1683 = local write "Set Strk"(1.0 ("Set Strk")) -> ()
        n1684 = local write "NORMAL LOAD"(200.0 ("NORMAL LOAD")) -> ()
        n1685 = local write "Set Temp"(60.0 ("Set Temp")) -> ()
        n1686 = local write "test time"(75.0 ("test time")) -> ()
        n1687 = local write "Set Hz"(50.0 ("Hz")) -> ()
        n1688 = local write "Set Rh"(53.0 ("Set Rh")) -> ()
      }
      frame "CEC F-096-A-06" {
        n1689 = local write "Set Strk"(1.0 ("Set Strk")) -> ()
        n1690 = local write "NORMAL LOAD"(200.0 ("NORMAL LOAD")) -> ()
        n1691 = local write "Set Temp"(60.0 ("Set Temp")) -> ()
        n1692 = local write "test time"(75.0 ("test time")) -> ()
        n1693 = local write "Set Hz"(50.0 ("Hz")) -> ()
        n1694 = local write "Set Rh"(53.0 ("Set Rh")) -> ()
      }
      frame "Custom" {
      }
    }
    n1695 = case shown="True" "Prog Due" {
      frame False {
      }
      frame True {
        n1696 = stacked-sequence {
          frame #0 {
            n1697 = Delete(path (use dialog)=path "C:/LAB-IQ/DUECOMPILE.bat" ("working directory")) -> ()  [unwired: 4 in, 3 out]
          }
          frame #1 {
            n1698 = disable-structure shown="Disabled" {
              frame Disabled {
                n1699 = local read "visa due"() -> (w2209:string)
                n1700 = Concatenate Strings("cmd.exe /c \"mode " ("command line"), w2209, ":1200,n,8,1\"\n" ("command line")) -> (w2214:string)
                n1701 = Concatenate Strings(w2214, "CD\\\nCD WinDucom\nTIMEOUT 1\n bossac.exe -i -d --port=" ("command line"), w2209, " -U false -e -w -v -b DUE.bin -R\n" ("command line"), "\r") -> (w2216:string)
                "concatenated string 2" <- w2216
                n1702 = call <vilib>:"Write Characters To File.vi"("append to file? (new file:F)"=FALSE, "character string"=w2216, "file path (dialog if empty)"=path "C:/LAB-IQ-NXT/DUECOMPILE.bat" ("working directory")) -> ()  [unwired: 2 in, 1 out]
              }
              frame Enabled {
              }
            }
          }
          frame #2 {
            # "C:\\LAB-IQ-NXT\\DUECOMPILE.bat"
            n1703 = disable-structure shown="Disabled" {
              frame Disabled {
                w2221 = "cmd.exe  /c \"C:\\LAB-IQ-NXT\\DUECOMPILE.bat\"" ("string")
                n1704 = call <vilib>:"System Exec.vi"("expected output size  (4096)"=u32 65535, "run minimized? (F)"=FALSE, "wait until completion? (T)"=TRUE ("run minimized? (F)"), "working directory"=path "C:/LAB-IQ-NXT", "standard input"=w2221, "command line"=w2221) -> ("error out"=w2220:errorcluster, "standard output"=→"String 44":string)  [unwired: 2 in, 2 out]
                "error out 4" <- w2220
                n1705 = flat-sequence {
                  tunnel: w2220 -> [_]
                  frame #0 {
                  }
                }
              }
              frame Enabled {
              }
            }
            n1706 = local write "Prog Due"(FALSE ("Prog Due")) -> ()
          }
        }
      }
    }
    n1707 = Or(x=w1628, y=w1626) -> (x .or. y?=w1627:bool)
    n1708 = case shown="\"About\"" w1625 {
      tunnel: [T20."Acquire" ("Main Tab") T20."Compare Files" ("Main Tab") T20."About" ("Main Tab")] -> w1638
      frame "Acquire", Default {
      }
      frame "Compare Files" {
      }
      frame "About" {
      }
    }
    n1709 = Or(x=w1632, y="OPEN") -> (x .or. y?=w1633:bool)
    n1710 = case shown="True" w1633 {
      tunnel: w1632 -> [_ w1773]
      frame False {
      }
      frame True {
        n1711 = stacked-sequence {
          tunnel: w1773 -> [_ w1840 _ _]
          frame #0 {
            w1789 = "  " ("String 6")
            n1712 = local write "OPEN"(FALSE ("open")) -> ()
            n1713 = local read "string1 2"() -> (w1777:string)
            n1714 = local read "string1 3"() -> (w1776:string)
            n1715 = local read "string1 4"() -> (w1775:string)
            n1716 = property on="OPEN" class="Bool (strict)"("Visible"=FALSE) -> ()  [unwired: 2 in, 2 out]
            n1717 = local write "String 6"(w1789) -> ()
            n1718 = local write "String 7"(w1789) -> ()
            n1719 = local write "String 8"(w1789) -> ()
            n1720 = local write "String 12"(w1789) -> ()
            n1721 = local read "OK Button 16"() -> (w1774:bool)
            n1722 = String To Path(string=w1777) -> (path=w1785:path)
            n1723 = String To Path(string=w1776) -> (path=w1784:path)
            n1724 = String To Path(string=w1775) -> (path=w1783:path)
            n1725 = case shown="True" w1774 {
              tunnel: [w1790 w1791] -> w1778
              frame False {
                n1726 = local read "string1"() -> (w1790:string)
              }
              frame True {
                n1727 = local read "String Indicator 4"() -> (w1791:string)
              }
            }
            n1728 = Open/Create/Replace File "Open File"(file path (use dialog)=w1785) -> (refnum out=w1781:refnum<file>)  [unwired: 5 in, 2 out]
            n1729 = Open/Create/Replace File "Open File"(file path (use dialog)=w1784) -> (refnum out=w1780:refnum<file>)  [unwired: 5 in, 2 out]
            n1730 = Open/Create/Replace File "Open File"(file path (use dialog)=w1783) -> (refnum out=w1779:refnum<file>)  [unwired: 5 in, 2 out]
            n1731 = while {
              tunnel: w1781 -> [w1803]
              i -> [w1799]
              stop <- w1798 continue-if-true
              (unwired) TRUE ("line mode (F)")
              n1732 = Read from Text File "Read File"(file (use dialog)=w1803) -> (text=w1800:string)  [unwired: 3 in, 3 out]
              n1733 = local write "Numeric 11"(w1799) -> ()
              n1734 = String Length(string=w1800) -> (length=w1802:i32)
              n1735 = Greater?(x=w1802, y=1) -> (0:w1798:bool)
            }
            n1736 = while {
              tunnel: w1780 -> [w1809]
              i -> [w1805]
              stop <- w1804 continue-if-true
              (unwired) TRUE ("line mode (F)")
              n1737 = Read from Text File "Read File"(file (use dialog)=w1809) -> (text=w1806:string)  [unwired: 3 in, 3 out]
              n1738 = local write "Numeric 12"(w1805) -> ()
              n1739 = String Length(string=w1806) -> (length=w1808:i32)
              n1740 = Greater?(x=w1808, y=1) -> (0:w1804:bool)
            }
            n1741 = while {
              tunnel: w1779 -> [w1815]
              i -> [w1811]
              stop <- w1810 continue-if-true
              (unwired) TRUE ("line mode (F)")
              n1742 = Read from Text File "Read File"(file (use dialog)=w1815) -> (text=w1812:string)  [unwired: 3 in, 3 out]
              n1743 = local write "Numeric 13"(w1811) -> ()
              n1744 = String Length(string=w1812) -> (length=w1814:i32)
              n1745 = Greater?(x=w1814, y=1) -> (0:w1810:bool)
            }
            n1746 = String To Path(string=w1778) -> (path=w1786:path)
            n1747 = Open/Create/Replace File "Open File"(file path (use dialog)=w1786) -> (refnum out=w1782:refnum<file>)  [unwired: 5 in, 2 out]
            n1748 = while {
              tunnel: w1782 -> [w1797]
              i -> [w1793]
              stop <- w1792 continue-if-true
              (unwired) TRUE ("line mode (F)")
              n1749 = Read from Text File "Read File"(file (use dialog)=w1797) -> (text=w1794:string)  [unwired: 3 in, 3 out]
              n1750 = local write "Numeric 8"(w1793) -> ()
              n1751 = String Length(string=w1794) -> (length=w1796:i32)
              n1752 = Greater?(x=w1796, y=1) -> (0:w1792:bool)
            }
          }
          frame #1 {
            w1967 = FALSE ("ACTUAL   MERGE")
            # "Sample Temp"
            # "ECR"
            # "COF"
            # "Time\nCOF\nFF\nTemp"
            n1753 = case shown="True" w1840 {
              tunnel: [w1987 w1988] -> w1841
              frame False {
                n1754 = local read "string1"() -> (w1987:string)
              }
              frame True {
                n1755 = local read "String Indicator 4"() -> (w1988:string)
              }
            }
            n1756 = local read "string1 3"() -> (w1885:string)
            n1757 = String To Path(string=w1841) -> (path=w1972:path)
            n1758 = String To Path(string=w1885) -> (path=w1983:path)
            n1759 = local read "Numeric 12"() -> (w1969:i32)
            n1760 = local read "Numeric 8"() -> (w1971:i32)
            n1761 = local read "string1 2"() -> (w1886:string)
            n1762 = local read "string1 4"() -> (w1884:string)
            n1763 = Open/Create/Replace File "Open File"(file path (use dialog)=w1972) -> (refnum out=w1986:refnum<file>, error out=w1985:errorcluster)  [unwired: 5 in, 1 out]
            n1764 = Open/Create/Replace File "Open File"(file path (use dialog)=w1983) -> (refnum out=w1979:refnum<file>, error out=w1980:errorcluster)  [unwired: 5 in, 1 out]
            n1765 = for {
              N: w1971 -> [_]
              tunnel: w1986 -> [w2134]
              tunnel: w1985 -> [w2133]
              tunnel: [w2123] -> w1898 mode=indexing
              tunnel: [w2121] -> w1955 mode=indexing
              tunnel: [w2122] -> w1950 mode=indexing
              tunnel: w1967 -> [_]
              tunnel: [w2115] -> w1952 mode=indexing
              tunnel: [w2111] -> w1921 mode=indexing
              tunnel: [w2107] -> w1896 mode=indexing
              tunnel: [w2103] -> w1877 mode=indexing
              tunnel: [w2098] -> w1837 mode=indexing
              (unwired) TRUE ("line mode (F)")
              # "freq"
              # "Stroke"
              # "Time"
              # "CoF"
              # "Humidity"
              # "Temp"
              # "Air Temp"
              # "ECR"
              n1766 = Read from Text File "Read File"(file (use dialog)=w2134, error in=w2133) -> (text=w2099:string)  [unwired: 2 in, 3 out]
              n1767 = local write "String 6"(w2099) -> ()
              n1768 = String Subset(string=w2099, offset (0)=0, length (rest)=14 ("length (rest)")) -> (substring=w2127:string)
              n1769 = String Subset(string=w2099, offset (0)=35, length (rest)=9 ("length (rest)")) -> (substring=w2124:string)
              n1770 = String Subset(string=w2099, offset (0)=15, length (rest)=9 ("length (rest)")) -> (substring=w2130:string)
              n1771 = Fract/Exp String To Number(string=w2127) -> (number=w2123:dbl)  [unwired: 3 in, 1 out]
              n1772 = Fract/Exp String To Number(string=w2124) -> (number=w2122:dbl)  [unwired: 3 in, 1 out]
              n1773 = Fract/Exp String To Number(string=w2130) -> (number=w2121:dbl)  [unwired: 3 in, 1 out]
              n1774 = String Subset(string=w2099, offset (0)=85, length (rest)=9 ("length (rest)")) -> (substring=w2100:string)
              n1775 = String Subset(string=w2099, offset (0)=25, length (rest)=9 ("length (rest)")) -> (substring=w2106:string)
              n1776 = String Subset(string=w2099, offset (0)=55, length (rest)=9 ("length (rest)")) -> (substring=w2108:string)
              n1777 = String Subset(string=w2099, offset (0)=45, length (rest)=9 ("length (rest)")) -> (substring=w2114:string)
              n1778 = String Subset(string=w2099, offset (0)=65, length (rest)=9 ("length (rest)")) -> (substring=w2120:string)
              n1779 = Fract/Exp String To Number(string=w2106) -> (number=w2103:dbl)  [unwired: 3 in, 1 out]
              n1780 = Fract/Exp String To Number(string=w2100) -> (number=w2098:dbl)  [unwired: 3 in, 1 out]
              n1781 = Fract/Exp String To Number(string=w2108) -> (number=w2107:dbl)  [unwired: 3 in, 1 out]
              n1782 = Fract/Exp String To Number(string=w2114) -> (number=w2111:dbl)  [unwired: 3 in, 1 out]
              n1783 = Fract/Exp String To Number(string=w2120) -> (number=w2117:dbl)  [unwired: 3 in, 1 out]
              n1784 = Add(x=w2117, y=0.0) -> (x+y=w2115:dbl)
            }
            n1785 = for {
              N: w1969 -> [_]
              tunnel: w1980 -> [w2060]
              tunnel: w1979 -> [w2059]
              tunnel: [w2049] -> w1938 mode=indexing
              tunnel: [w2047] -> w1936 mode=indexing
              tunnel: [w2048] -> w1932 mode=indexing
              tunnel: w1967 -> [_]
              tunnel: [w2041] -> w1934 mode=indexing
              tunnel: [w2037] -> w1916 mode=indexing
              tunnel: [w2033] -> w1892 mode=indexing
              tunnel: [w2030] -> w1873 mode=indexing
              tunnel: [w2026] -> w1832 mode=indexing
              (unwired) 9 ("length (rest)")
              (unwired) 9 ("length (rest)")
              (unwired) TRUE ("line mode (F)")
              n1786 = Read from Text File "Read File"(file (use dialog)=w2059, error in=w2060) -> (text=w2027:string)  [unwired: 2 in, 3 out]
              n1787 = local write "String 8"(w2027) -> ()
              n1788 = String Subset(string=w2027, offset (0)=85) -> (substring=w2029:string)  [unwired: 1 in]
              n1789 = String Subset(string=w2027, offset (0)=35, length (rest)=9 ("length (rest)")) -> (substring=w2050:string)
              n1790 = String Subset(string=w2027, offset (0)=55, length (rest)=9 ("length (rest)")) -> (substring=w2035:string)
              n1791 = String Subset(string=w2027, offset (0)=25) -> (substring=w2031:string)  [unwired: 1 in]
              n1792 = String Subset(string=w2027, offset (0)=15, length (rest)=9 ("length (rest)")) -> (substring=w2056:string)
              n1793 = String Subset(string=w2027, offset (0)=0, length (rest)=14 ("length (rest)")) -> (substring=w2053:string)
              n1794 = String Subset(string=w2027, offset (0)=45, length (rest)=9 ("length (rest)")) -> (substring=w2040:string)
              n1795 = String Subset(string=w2027, offset (0)=65, length (rest)=9 ("length (rest)")) -> (substring=w2046:string)
              n1796 = Fract/Exp String To Number(string=w2029) -> (number=w2026:dbl)  [unwired: 3 in, 1 out]
              n1797 = Fract/Exp String To Number(string=w2050) -> (number=w2048:dbl)  [unwired: 3 in, 1 out]
              n1798 = Fract/Exp String To Number(string=w2035) -> (number=w2033:dbl)  [unwired: 3 in, 1 out]
              n1799 = Fract/Exp String To Number(string=w2031) -> (number=w2030:dbl)  [unwired: 3 in, 1 out]
              n1800 = Fract/Exp String To Number(string=w2056) -> (number=w2047:dbl)  [unwired: 3 in, 1 out]
              n1801 = Fract/Exp String To Number(string=w2053) -> (number=w2049:dbl)  [unwired: 3 in, 1 out]
              n1802 = Fract/Exp String To Number(string=w2040) -> (number=w2037:dbl)  [unwired: 3 in, 1 out]
              n1803 = Fract/Exp String To Number(string=w2046) -> (number=w2043:dbl)  [unwired: 3 in, 1 out]
              n1804 = Add(x=w2043, y=0.0) -> (x+y=w2041:dbl)
            }
            n1805 = String To Path(string=w1886) -> (path=w1984:path)
            n1806 = String To Path(string=w1884) -> (path=w1978:path)
            n1807 = local read "Numeric 11"() -> (w1968:i32)
            n1808 = local read "Numeric 13"() -> (w1970:i32)
            n1809 = Open/Create/Replace File "Open File"(file path (use dialog)=w1984) -> (refnum out=w1982:refnum<file>, error out=w1981:errorcluster)  [unwired: 5 in, 1 out]
            n1810 = Open/Create/Replace File "Open File"(file path (use dialog)=w1978) -> (refnum out=w1977:refnum<file>, error out=w1976:errorcluster)  [unwired: 5 in, 1 out]
            n1811 = for {
              N: w1968 -> [_]
              tunnel: w1982 -> [w2097]
              tunnel: w1981 -> [w2096]
              tunnel: [w2086] -> w1948 mode=indexing
              tunnel: [w2084] -> w1946 mode=indexing
              tunnel: [w2085] -> w1941 mode=indexing
              tunnel: w1967 -> [_]
              tunnel: [w2078] -> w1943 mode=indexing
